vi "crc16.vi"(1 "Message":string) -> (0 "crc 16":string)   [LabVIEW 2023, in "Laser_Ethernet.lvclass"]
uses:
  Laser_Ethernet.lvclass
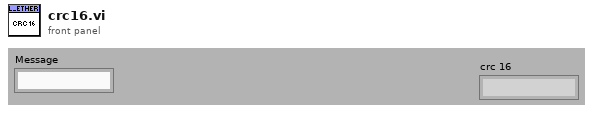
[diagram p1: front panel]
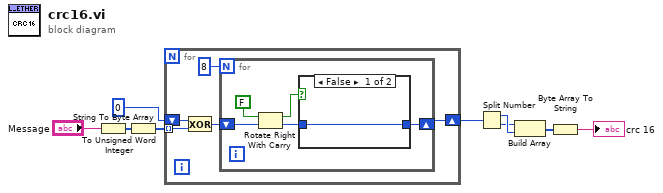
[diagram p0: block diagram]
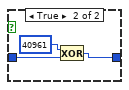
[diagram p2: hidden frame]
diagram:
  n1 = String To Byte Array(string="Message") -> (unsigned byte array=w3:u8[])
  n2 = To Unsigned Word Integer(number=w3) -> (unsigned 16bit integer=w4:u16[])
  n3 = for {
    shift-right: [w11] -> w2
    shift-left: u16 0 -> [w12]
    tunnel: w4 -> [w10] mode=indexing
    n4 = Exclusive Or(1:w10, 2:w12) -> (0:w13:u16)
    n5 = for {
      N: 8 -> [_]
      shift-right: [w18] -> w11
      shift-left: w13 -> [w17]
      n6 = Rotate Right With Carry(2:w17, 3:FALSE ("Übertrag")) -> (0:w19:u16, 1:w16:bool)
      n7 = case shown="False" w16 {
        tunnel: w19 -> [w20 w22]
        tunnel: [w20 w21] -> w18
        frame False {
        }
        frame True {
          n8 = Exclusive Or(1:w22, 2:u16 40961) -> (0:w21:u16)
        }
      }
    }
  }
  n9 = Split Number(x=w2) -> (hi(x)=w6:u8, lo(x)=w5:u8)
  n10 = Build Array(w5, w6) -> (w7:u8[])
  n11 = Byte Array To String(unsigned byte array=w7) -> (string=→"crc 16":string)
